vi "HostVI.vi"() -> ()   [LabVIEW 2014]
uses:
  Controls/State.ctl
  <vilib>/rvi/interface/RandomDataEmulation/nirviRandomDataOpen.vi
  <vilib>/rvi/interface/common/niFpgaCacheSessionInfoDynamic.vi
  <vilib>/rvi/interface/common/niFpgaWaitOnOcc.vi
  <vilib>/Utility/error.llb/Error Cluster From Error Code.vi
  <vilib>/rvi/errors/niLvFpgaAdjustHostInterfaceError.vi
  <vilib>/FPGAPlugInAG/Dynamic/niLvFpga_Close_Dynamic.vi
  <vilib>/rvi/interface/nirviOpenFPGA/nirviOpenFPGA.xnode
  FPGA_VI.vi
  <vilib>/rvi/interface/nirviMethod/nirviMethod.xnode
  <vilib>/rvi/interface/nirviReadWriteControl/nirviReadWriteControl.xnode
  <vilib>/rvi/interface/nirviCloseFPGA/nirviCloseFPGA.xnode
  <vilib>/rvi/interface/Simulation/niFpgaSimulationCallBeginRW.vi
  <vilib>/FPGAPlugInAG/Dynamic/niLvFpga_ReadFifo_Dynamic.vi
  <vilib>/rvi/errors/niLvFpgaMergeErrorWithErrorCode.vi
  <vilib>/FPGAPlugInAG/Dynamic/niLvFpga_ConfigureFifo_Dynamic.vi
  <vilib>/FPGAPlugInAG/Dynamic/niLvFpga_StartFifo_Dynamic.vi
  NiFpgaLv.dll
panel:
  out "error out":errorcluster
  out "Channels 12-15":dbl[][](graph)
  out "Channels 8-11":dbl[][](graph)
  out "Channels 4-7":dbl[][](graph)
  out "Channels 0-3":dbl[][](graph)
  in  "stop":bool
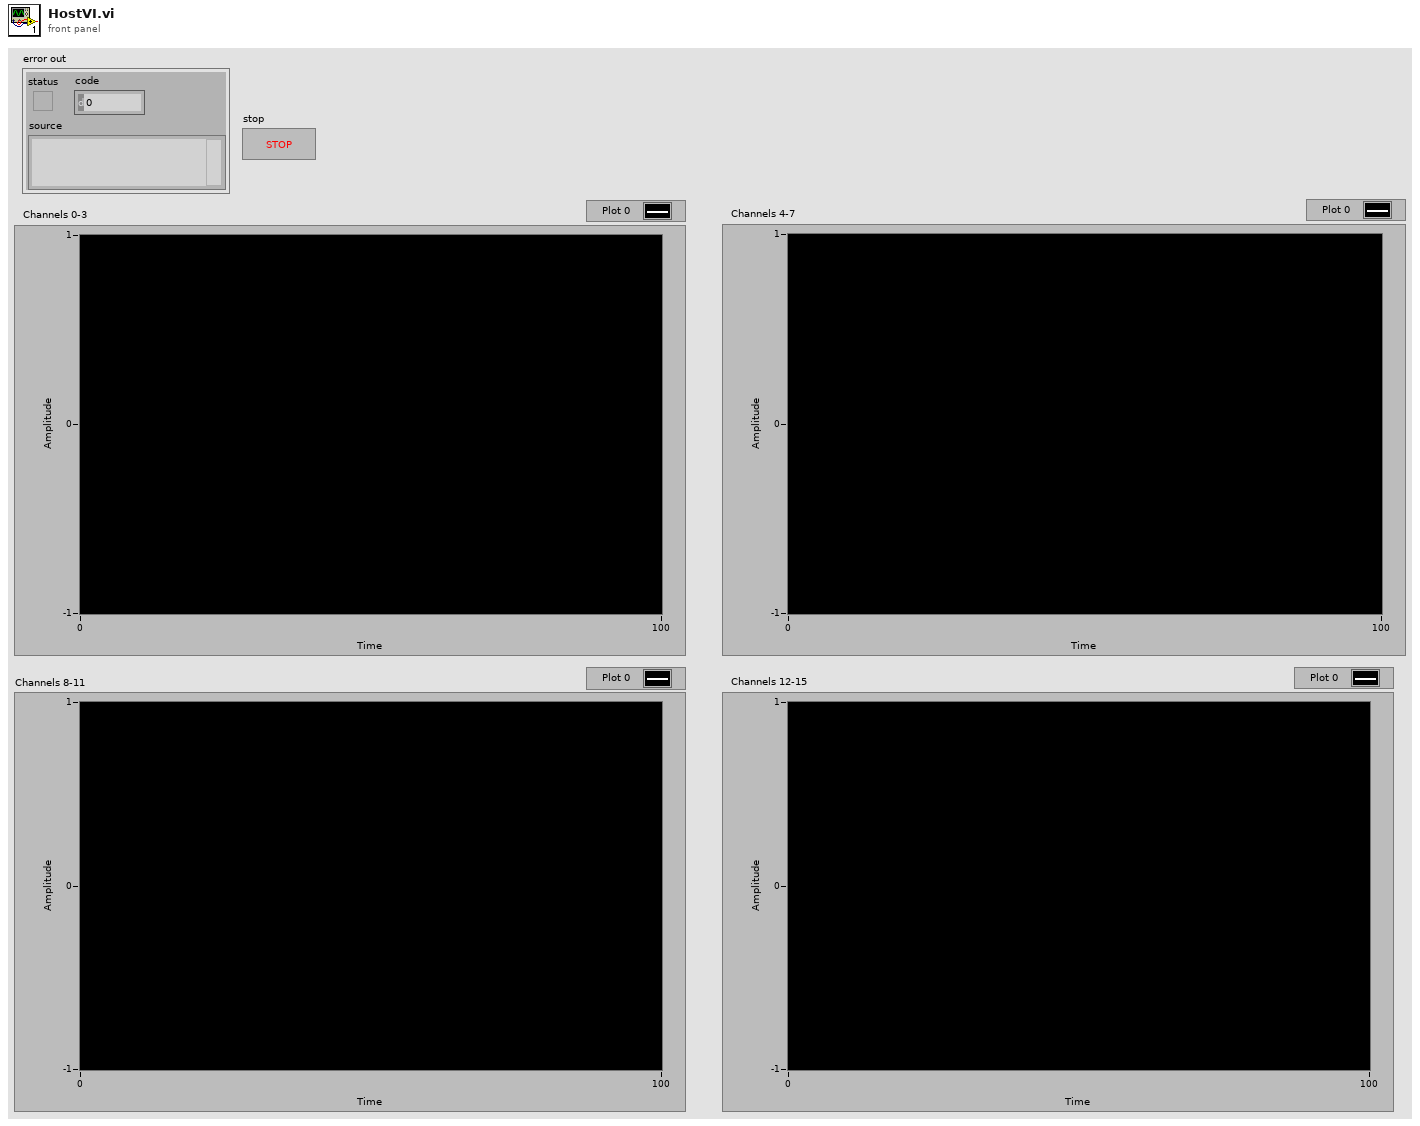
[diagram p1: front panel]
types:
  T1 = typedef "State.ctl" = enum16{"Trigger", "Fetch Data DRAM 0", "Fetch Data DRAM 1", "Graph Data", "Idle"}
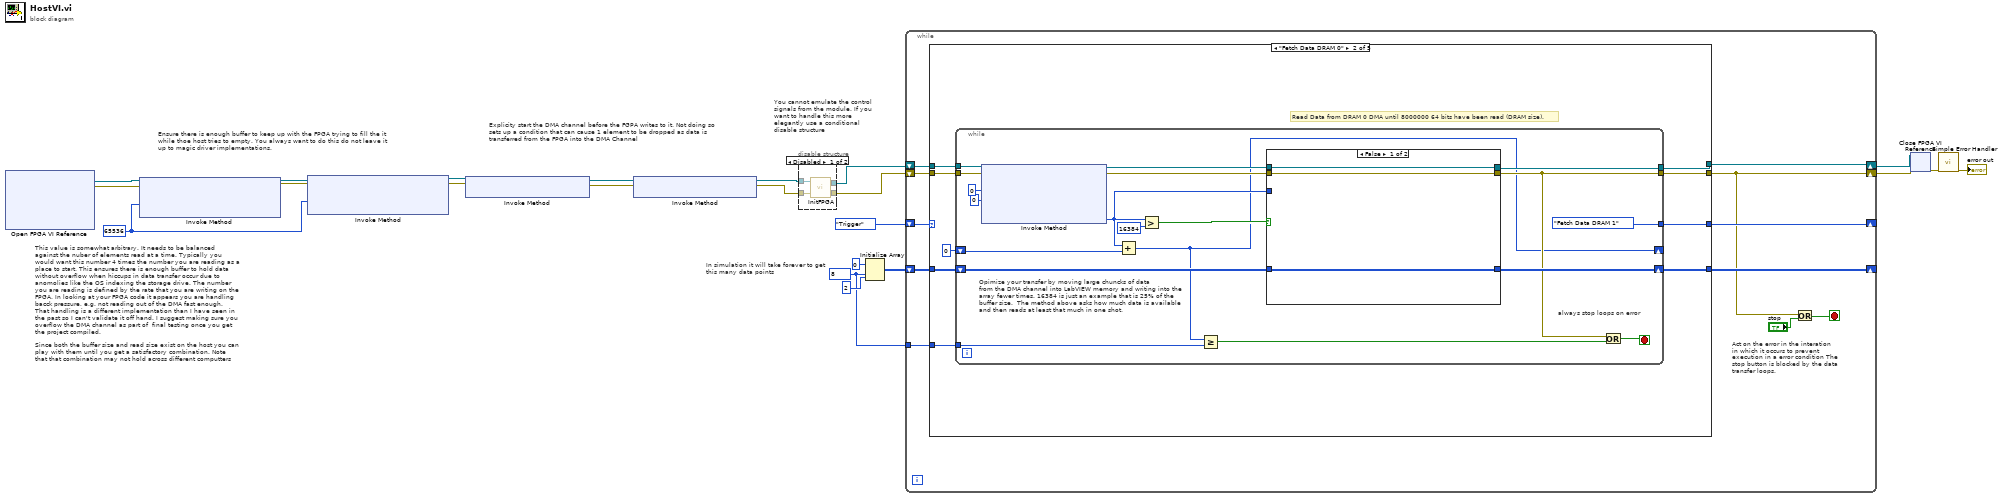
[diagram p0: block diagram]
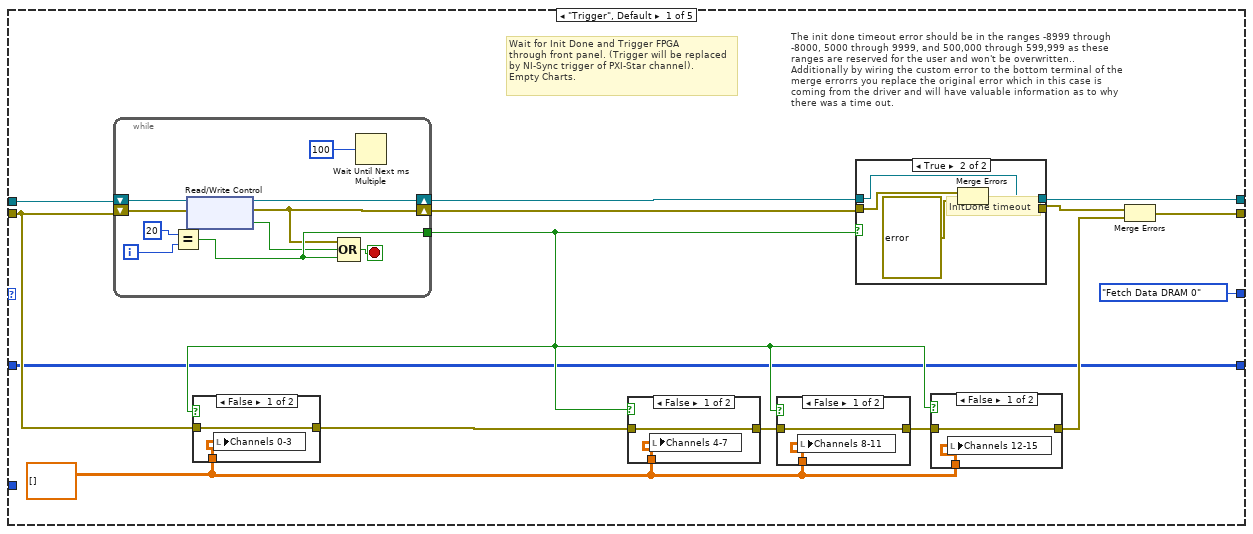
[diagram p3: hidden frame]
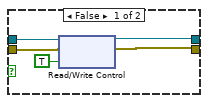
[diagram p4: hidden frame]
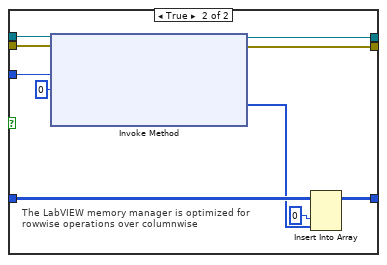
[diagram p9: hidden frame]
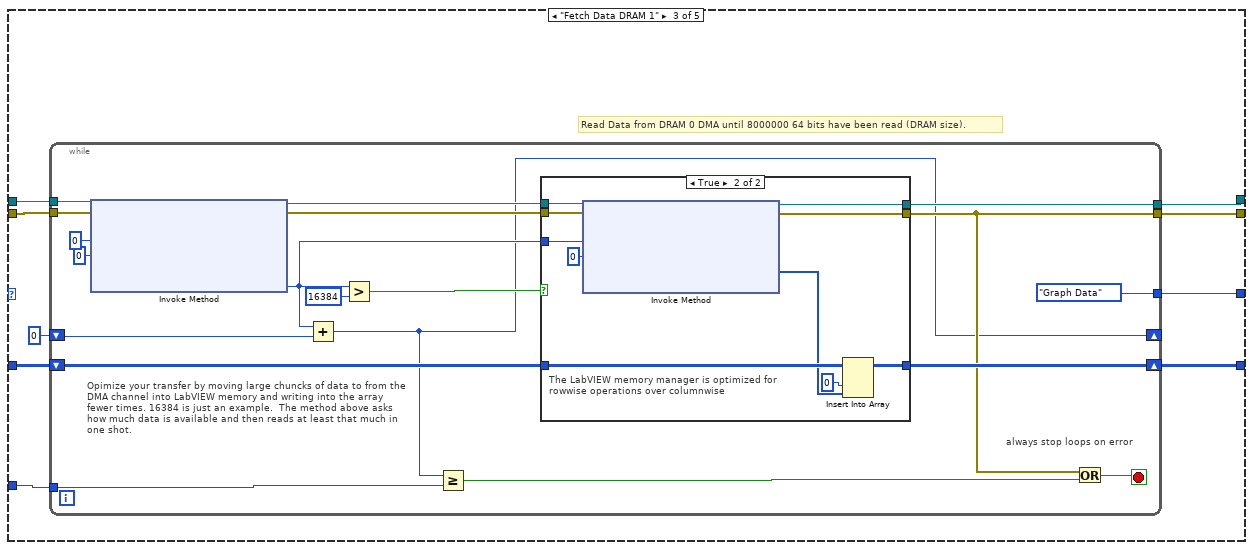
[diagram p10: hidden frame]
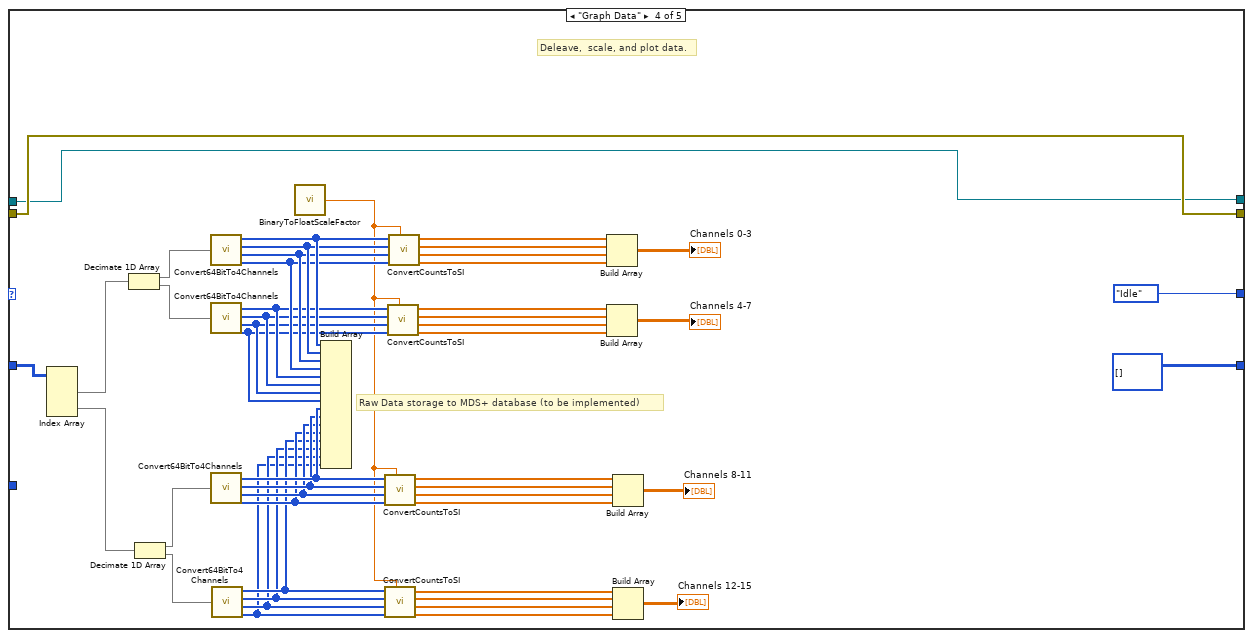
[diagram p12: hidden frame]
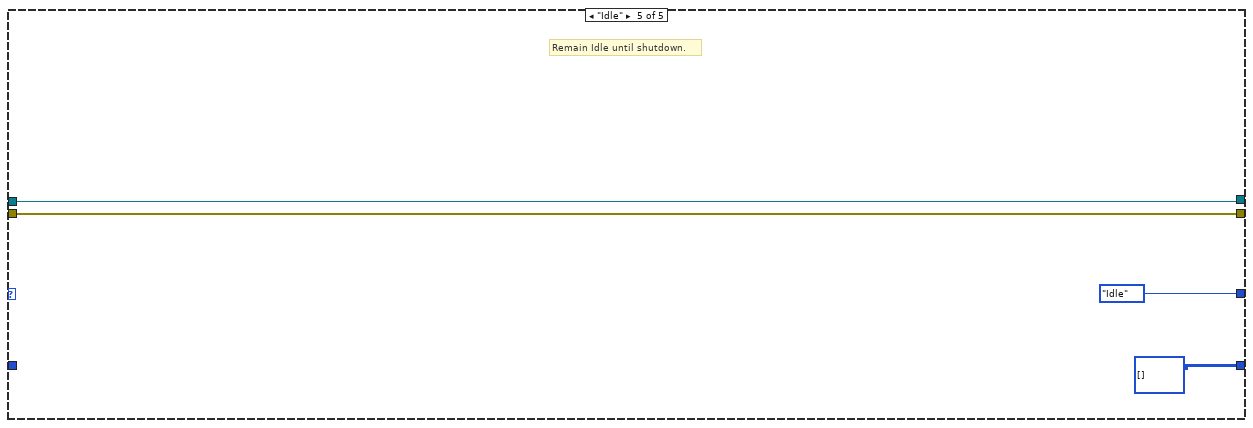
[diagram p13: hidden frame]
diagram:
  w1 = u32 65536 ("Requested Depth")
  w16 = 8 ("dimension size")
  # "You cannot emulate the control signals from the module. If you want to handle this more elegantly use a conditional disable structure"
  # "In simulation it will take forever to get this many data points"
  # "This value is somewhat arbitrary. It needs to be balanced against the nuber of elements read at a time. Typically you would want this number 4 times the number you are reading as a place to start. This ensures there is enough buffer to hold data without overflow when hiccups in data transfer occur due to anomolies like the OS indexing the storage drive. The number you are reading is defined by the rate that you are writing on the FPGA. In looking at your FPGA code it appears you are handling bacck pressure, e.g. not reading out of the DMA fast enough. That handling is a different implementation than I have seen in the past so I can't validate it off hand. I suggest making sure you overflow the DMA channel as part of  final testing once you get the project compiled. \n\nSince both the buffer size and read size exist on the host you can play with them until you get a satisfactory combination. Note that that combination may not hold across different computters"
  # "Explicity start the DMA channel before the FGPA writes to it. Not doing so sets up a condition that can cause 1 element to be dropped as data is transferred from the FPGA into the DMA Channel"
  # "Ensure there is enough buffer to keep up with the FPGA trying to fill the it while thoe host tries to empty. You always want to do this do not leave it up to magic driver implementations."
  n1 = xnode "Open FPGA VI Reference"() -> ("FPGA VI Reference Out"=w11:refnum<k20>, "error out"=w10:errorcluster)  [unwired: 2 in]
  n2 = xnode "Invoke Method"("FPGA VI Reference In"=w11, "error in"=w10, "Requested Depth"=w1) -> ("FPGA VI Reference Out"=w9:refnum<k20>, "error out"=w8:errorcluster)  [unwired: 1 out]
  n3 = xnode "Invoke Method"("FPGA VI Reference In"=w9, "error in"=w8, "Requested Depth"=w1) -> ("FPGA VI Reference Out"=w7:refnum<k20>, "error out"=w6:errorcluster)  [unwired: 1 out]
  n4 = xnode "Invoke Method"("FPGA VI Reference In"=w7, "error in"=w6) -> ("FPGA VI Reference Out"=w5:refnum<k20>, "error out"=w4:errorcluster)
  n5 = xnode "Invoke Method"("FPGA VI Reference In"=w5, "error in"=w4) -> ("FPGA VI Reference Out"=w3:refnum<k20>, "error out"=w2:errorcluster)
  n6 = disable-structure shown="Disabled" {
    disable-tunnel: [w26 w27] -> w20
    disable-tunnel: w3 -> [w25 w28]
    disable-tunnel: [w24 w28] -> w12
    disable-tunnel: w2 -> [w23 w27]
    frame Disabled {
      n7 = call "InitFPGA.vi"("error in"=w23, "FPGA VI Reference In"=w25) -> ("error out"=w26:errorcluster, "FPGA VI Reference Out"=w24:refnum<k20>)
    }
    frame Enabled {
    }
  }
  n8 = Initialize Array(u64 0 ("element"), w16, 2 ("dimension size")) -> (w17:u64[][])
  n9 = while {
    shift-right: [w29] -> w14
    shift-left: w20 -> [w33]
    shift-right: [w36] -> _
    shift-left: w17 -> [w38]
    tunnel: w16 -> [w37]
    shift-right: [w34] -> _
    shift-left: State."Trigger" -> [w35]
    shift-right: [w30] -> w13
    shift-left: w12 -> [w31]
    stop <- w39 stop-if-true
    # "Act on the error in the interation in which it occurs to prevent execution in a error condition The stop button is blocked by the data transfer loops."
    n10 = case shown="\"Fetch Data DRAM 0\"" w35 {
      tunnel: w31 -> [w48 w94 w135 w205 w216]
      tunnel: w33 -> [w47 w93 w134 w208 w219]
      tunnel: [w43 w92 w133 w208 w219] -> w29
      tunnel: w38 -> [w42 w91 w132 w215 _]
      tunnel: w37 -> [_ w90 w131 _ _]
      tunnel: [w42 w89 w130 u64[][] [] u64[][] []] -> w36
      tunnel: [State."Fetch Data DRAM 0" w88 w129 State."Idle" State."Idle"] -> w34
      tunnel: [w41 w87 w128 w205 w216] -> w30
      frame "Trigger", Default {
        w53 = dbl[][] [] ("ADC A Graph")
        # "The init done timeout error should be in the ranges -8999 through -8000, 5000 through 9999, and 500,000 through 599,999 as these ranges are reserved for the user and won't be overwritten.. Additionally by wiring the custom error to the bottom terminal of the merge errorrs you replace the original error which in this case is coming from the driver and will have valuable information as to why there was a time out."
        # "Wait for Init Done and Trigger FPGA\nthrough front panel. (Trigger will be replaced\nby NI-Sync trigger of PXI-Star channel).\nEmpty Charts."
        n11 = while {
          tunnel: [w58] -> w44
          shift-right: [w60] -> w49
          shift-left: w48 -> [w64]
          shift-right: [w55] -> w46
          shift-left: w47 -> [w56]
          i -> [w62]
          stop <- w59 stop-if-true
          n12 = Equal?(x=20, y=w62) -> (x = y?=w58:bool)
          n13 = xnode "Read/Write Control"("FPGA VI Reference In"=w64, "error in"=w56) -> ("FPGA VI Reference Out"=w60:refnum<k20>, "error out"=w55:errorcluster, "Init Done"=w57:bool)
          n14 = Compound Arithmetic op=OR(w55, w57, w58) -> (w59:bool)
          n15 = Wait Until Next ms Multiple(millisecond multiple=u32 100) -> ()  [unwired: 1 out]
        }
        n16 = case shown="False" w44 {
          tunnel: w47 -> [w83 w85]
          tunnel: w53 -> [w84 _]
          tunnel: [w83 w85] -> w52
          frame False {
            n17 = local write "Channels 0-3"(w84) -> ()
          }
          frame True {
          }
        }
        n18 = case shown="False" w44 {
          tunnel: w53 -> [w81 _]
          tunnel: w52 -> [w80 w82]
          tunnel: [w80 w82] -> w51
          frame False {
            n19 = local write "Channels 4-7"(w81) -> ()
          }
          frame True {
          }
        }
        n20 = case shown="False" w44 {
          tunnel: w53 -> [w78 _]
          tunnel: w51 -> [w77 w79]
          tunnel: [w77 w79] -> w50
          frame False {
            n21 = local write "Channels 8-11"(w78) -> ()
          }
          frame True {
          }
        }
        n22 = case shown="True" w44 {
          tunnel: [w67 w71] -> w41
          tunnel: w49 -> [w69 w71]
          tunnel: w46 -> [w68 w70]
          tunnel: [w66 w73] -> w40
          frame False {
            n23 = xnode "Read/Write Control"("FPGA VI Reference In"=w69, "error in"=w68, "Trigger"=TRUE) -> ("FPGA VI Reference Out"=w67:refnum<k20>, "error out"=w66:errorcluster)
          }
          frame True {
            # "InitDone timeout"
            n24 = Merge Errors(w70, errorcluster {"status"=TRUE, "code"=-1, "source"="The IO Module CLIP was not ready. If you are using any external clocks, make sure they are connected and within the supported specifications."} ("error in")) -> (w73:errorcluster)
          }
        }
        n25 = case shown="False" w44 {
          tunnel: [w74 w76] -> w54
          tunnel: w53 -> [w75 _]
          tunnel: w50 -> [w74 w76]
          frame False {
            n26 = local write "Channels 12-15"(w75) -> ()
          }
          frame True {
          }
        }
        n27 = Merge Errors(w40, w54) -> (w43:errorcluster)
      }
      frame "Fetch Data DRAM 0" {
        # "Read Data from DRAM 0 DMA until 8000000 64 bits have been read (DRAM size)."
        n28 = while {
          tunnel: w94 -> [w113]
          tunnel: w93 -> [w111]
          tunnel: [w98] -> w92
          shift-right: [w107] -> w89
          shift-left: w91 -> [w108]
          tunnel: w90 -> [w101]
          tunnel: [State."Fetch Data DRAM 1"] -> w88
          tunnel: [w105] -> w87
          shift-right: [w95] -> _
          shift-left: u32 0 -> [w103]
          stop <- w97 stop-if-true
          # "always stop loops on error"
          # "Opimize your transfer by moving large chuncks of data \nfrom the DMA channel into LabVIEW memory and writing into the array fewer times. 16384 is just an example that is 25% of the buffer size.  The method above asks how much data is available and then reads at least that much in one shot."
          n29 = xnode "Invoke Method"("FPGA VI Reference In"=w113, "error in"=w111, "Number of Elements"=u32 0, "Timeout (ms)"=0) -> ("FPGA VI Reference Out"=w109:refnum<k20>, "error out"=w110:errorcluster, "Elements Remaining"=w102:u32)  [unwired: 1 out]
          n30 = Add(x=w102, y=w103) -> (x+y=w95:u32)
          n31 = Greater?(x=w102, y=u32 16384) -> (0:w96:bool)
          n32 = Greater Or Equal?(x=w95, y=w101) -> (x >= y?=w99:bool)
          n33 = case shown="False" w96 {
            tunnel: w110 -> [w114 w126]
            tunnel: w109 -> [w115 w125]
            tunnel: w108 -> [w116 w124]
            tunnel: [w116 w121] -> w107
            tunnel: [w115 w120] -> w105
            tunnel: w102 -> [_ w119]
            tunnel: [w114 w118] -> w98
            frame False {
            }
            frame True {
              # "The LabVIEW memory manager is optimized for rowwise operations over columnwise"
              n34 = xnode "Invoke Method"("FPGA VI Reference In"=w125, "error in"=w126, "Number of Elements"=w119, "Timeout (ms)"=0) -> ("FPGA VI Reference Out"=w120:refnum<k20>, "error out"=w118:errorcluster, "Data"=w123:u64[])  [unwired: 1 out]
              n35 = Insert Into Array(array=w124, index (col)=0 ("disabled index (col)"), new element=w123) -> (w121:u64[][])  [unwired: 1 in]
            }
          }
          n36 = Or(x=w98, y=w99) -> (x .or. y?=w97:bool)
        }
      }
      frame "Fetch Data DRAM 1" {
        # "Read Data from DRAM 0 DMA until 8000000 64 bits have been read (DRAM size)."
        n37 = while {
          tunnel: w135 -> [w154]
          tunnel: w134 -> [w152]
          tunnel: [w139] -> w133
          shift-right: [w148] -> w130
          shift-left: w132 -> [w149]
          tunnel: w131 -> [w142]
          tunnel: [State."Graph Data"] -> w129
          tunnel: [w146] -> w128
          shift-right: [w136] -> _
          shift-left: u32 0 -> [w144]
          stop <- w138 stop-if-true
          # "always stop loops on error"
          # "Opimize your transfer by moving large chuncks of data to from the DMA channel into LabVIEW memory and writing into the array fewer times. 16384 is just an example.  The method above asks how much data is available and then reads at least that much in one shot."
          n38 = xnode "Invoke Method"("FPGA VI Reference In"=w154, "error in"=w152, "Number of Elements"=u32 0, "Timeout (ms)"=0) -> ("FPGA VI Reference Out"=w150:refnum<k20>, "error out"=w151:errorcluster, "Elements Remaining"=w143:u32)  [unwired: 1 out]
          n39 = Add(x=w143, y=w144) -> (x+y=w136:u32)
          n40 = Greater?(x=w143, y=u32 16384) -> (0:w137:bool)
          n41 = Greater Or Equal?(x=w136, y=w142) -> (x >= y?=w140:bool)
          n42 = case shown="True" w137 {
            tunnel: w151 -> [w155 w167]
            tunnel: w150 -> [w156 w166]
            tunnel: w149 -> [w157 w165]
            tunnel: [w157 w162] -> w148
            tunnel: [w156 w161] -> w146
            tunnel: w143 -> [_ w160]
            tunnel: [w155 w159] -> w139
            frame False {
            }
            frame True {
              # "The LabVIEW memory manager is optimized for rowwise operations over columnwise"
              n43 = xnode "Invoke Method"("FPGA VI Reference In"=w166, "error in"=w167, "Number of Elements"=w160, "Timeout (ms)"=0) -> ("FPGA VI Reference Out"=w161:refnum<k20>, "error out"=w159:errorcluster, "Data"=w164:u64[])  [unwired: 1 out]
              n44 = Insert Into Array(array=w165, index (col)=0 ("disabled index (col)"), new element=w164) -> (w162:u64[][])  [unwired: 1 in]
            }
          }
          n45 = Or(x=w139, y=w140) -> (x .or. y?=w138:bool)
        }
      }
      frame "Graph Data" {
        # "Raw Data storage to MDS+ database (to be implemented)"
        # "Deleave,  scale, and plot data."
        n46 = Index Array(array=w215) -> (element #1=w214:u64[], element #2=w213:u64[])  [unwired: 4 in]
        n47 = Decimate 1D Array(w214) -> (w203:u64[], w204:u64[])
        n48 = Decimate 1D Array(w213) -> (w202:u64[], w201:u64[])
        n49 = call "Convert64BitTo4Channels.vi"("Interleaved Count Array"=w203) -> ("decimated array 0"=w200:i16[], "decimated array 1"=w199:i16[], "decimated array 2"=w198:i16[], "decimated array 3"=w197:i16[])
        n50 = call "Convert64BitTo4Channels.vi"("Interleaved Count Array"=w204) -> ("decimated array 0"=w196:i16[], "decimated array 1"=w195:i16[], "decimated array 2"=w194:i16[], "decimated array 3"=w193:i16[])
        n51 = call "Convert64BitTo4Channels.vi"("Interleaved Count Array"=w202) -> ("decimated array 0"=w192:i16[], "decimated array 1"=w191:i16[], "decimated array 2"=w190:i16[], "decimated array 3"=w189:i16[])
        n52 = call "Convert64BitTo4Channels.vi"("Interleaved Count Array"=w201) -> ("decimated array 0"=w188:i16[], "decimated array 1"=w187:i16[], "decimated array 2"=w186:i16[], "decimated array 3"=w185:i16[])
        n53 = call "BinaryToFloatScaleFactor.vi"() -> ("Scale Factor"=w168:dbl)  [unwired: 2 in]
        n54 = Build Array(w200, w199, w198, w197, w196, w195, w194, w193, w192, w191, w190, w189, w188, w187, w186, w185) -> ()  [unwired: 1 out]
        n55 = call "ConvertCountsToSI.vi"("Scale Factor"=w168, "Count Array 3"=w189, "Count Array 2"=w190, "Count Array 1"=w191, "Count Array 0"=w192) -> ("SI Array 3"=w177:dbl[], "SI Array 2"=w178:dbl[], "SI Array 1"=w179:dbl[], "SI Array 0"=w180:dbl[])  [unwired: 3 in]
        n56 = call "ConvertCountsToSI.vi"("Scale Factor"=w168, "Count Array 3"=w185, "Count Array 2"=w186, "Count Array 1"=w187, "Count Array 0"=w188) -> ("SI Array 3"=w181:dbl[], "SI Array 2"=w182:dbl[], "SI Array 1"=w183:dbl[], "SI Array 0"=w184:dbl[])  [unwired: 3 in]
        n57 = call "ConvertCountsToSI.vi"("Scale Factor"=w168, "Count Array 3"=w193, "Count Array 2"=w194, "Count Array 1"=w195, "Count Array 0"=w196) -> ("SI Array 3"=w173:dbl[], "SI Array 2"=w174:dbl[], "SI Array 1"=w175:dbl[], "SI Array 0"=w176:dbl[])  [unwired: 3 in]
        n58 = call "ConvertCountsToSI.vi"("Scale Factor"=w168, "Count Array 3"=w197, "Count Array 2"=w198, "Count Array 1"=w199, "Count Array 0"=w200) -> ("SI Array 3"=w169:dbl[], "SI Array 2"=w170:dbl[], "SI Array 1"=w171:dbl[], "SI Array 0"=w172:dbl[])  [unwired: 3 in]
        n59 = Build Array(w172, w171, w170, w169) -> (→"Channels 0-3":dbl[][])
        n60 = Build Array(w176, w175, w174, w173) -> (→"Channels 4-7":dbl[][])
        n61 = Build Array(w180, w179, w178, w177) -> (→"Channels 8-11":dbl[][])
        n62 = Build Array(w184, w183, w182, w181) -> (→"Channels 12-15":dbl[][])
      }
      frame "Idle" {
        # "Remain Idle until shutdown."
      }
    }
    n63 = Or(x=w29, y="stop") -> (x .or. y?=w39:bool)
  }
  n64 = xnode "Close FPGA VI Reference"("FPGA VI Reference In"=w13, "error in"=w14) -> ("error out"=w22:errorcluster)
  n65 = call <vilib>:"Simple Error Handler.vi"("error in (no error)"=w22) -> ("error out"=→"error out":errorcluster)  [unwired: 1 in, 7 out]
